vi "Open Form.vi"(8 "error in (no error)":errorcluster, 10 "Panel Form Controller":refnum<class "Panel Form Controller.lvclass">, 11 "Form Model in":refnum<class "Form Model.lvclass">) -> (0 "error out":errorcluster, 3 "Form Model out":refnum<class "Form Model.lvclass">)   [LabVIEW 2020, in "Form Model.lvlib" / "Form Model.lvclass"]
uses:
  Form Model.lvclass
  C:/Program Files (x86)/National Instruments/LabVIEW 2020/vi.lib/ActorFramework/Actor/Actor.lvclass
  Forms Controller/Form Controller/Panel Form Controller.lvclass
  <vilib>/ActorFramework/Actor/Actor.lvclass/Actor.ctl
  Form Model.lvclass/Form Model.ctl
  Forms Server/Form Server Messages Messages/Open Form Msg/Open Form Msg.lvclass/Open Form Msg.ctl
  <vilib>/ActorFramework/Message Enqueuer/Message Enqueuer.lvclass/Message Enqueuer.ctl
  <vilib>/ActorFramework/Message Enqueuer/Enqueue.vi
  Forms Server/Form Server Messages Messages/Open Form Msg/Open Form Msg.lvclass
  C:/Program Files (x86)/National Instruments/LabVIEW 2020/vi.lib/ActorFramework/Message/Message.lvclass
  <vilib>/ActorFramework/Message Priority Queue/Priority Enqueue.vi
  Form Model Configuration/Form Model Configuration Class/Form Model Configuration.lvclass
  Form Model Interfaces/Model Panel Logic Interface/Model Panel Logic.lvclass
  <vilib>/ActorFramework/Actor/Actor.lvclass
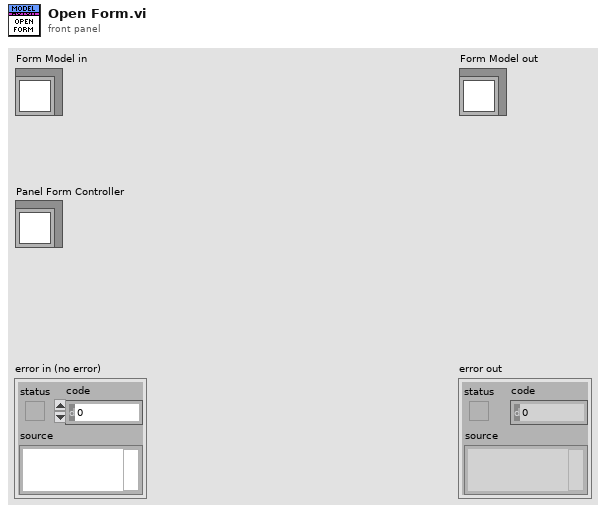
[diagram p1: front panel]
types:
  T1 = typedef "Form Server Interfaces.lvlib/Form ID.ctl" = cluster{"Name":string, "Panel type":string}
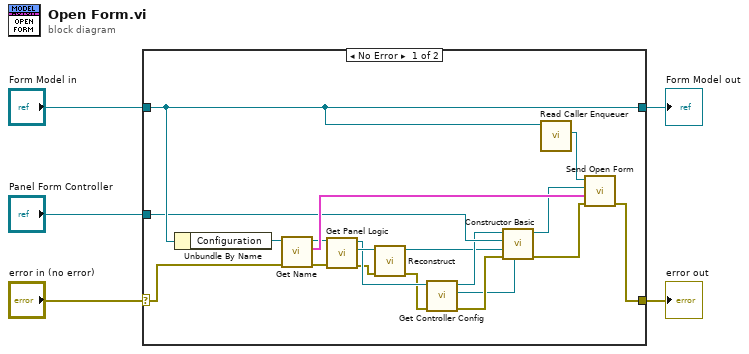
[diagram p0: block diagram]
diagram:
  n1 = case shown="No Error" "error in (no error)" {
    selector: "error in (no error)" -> [w15 w26]
    tunnel: "Form Model in" -> [w24 w25]
    tunnel: [w14 w26] -> w3
    tunnel: [w24 w25] -> w2
    tunnel: "Panel Form Controller" -> [w19 _]
    frame No Error {
      n2 = Unbundle By Name(w24) -> ("Configuration"=w22:refnum<class "Form Model Configuration.lvclass">)
      n3 = call-dynamic "Get Name.vi"("error in (no error)"=w15, "Form Configuration in"=w22) -> ("error out"=w11:errorcluster, "Form ID"=w21:T1, "Form Configuration out"=w12:refnum<class "Form Model Configuration.lvclass">)  [unwired: 7 in]
      n4 = call-dynamic "Get Panel Logic.vi"("error in (no error)"=w11, "Form Model Configuration in"=w12) -> ("error out"=w7:errorcluster, "Panel Logic"=w10:refnum<class "Model Panel Logic.lvclass">, "Form Model Configuration out"=w8:refnum<class "Form Model Configuration.lvclass">)  [unwired: 7 in]
      n5 = call-dynamic "Reconstruct.vi"("error in (no error)"=w7, "Model Panel Logic in"=w10) -> ("error out"=w6:errorcluster, "Model Panel Logic out"=w9:refnum<class "Model Panel Logic.lvclass">)  [unwired: 8 in]
      n6 = call-dynamic "Get Controller Config.vi"("error in (no error)"=w6, "Form Model Configuration in"=w8) -> ("error out"=w17:errorcluster, "Controller config"=w13:refnum<class "Panel Form Controller Configuration.lvclass">, "Form Model Configuration out"=w18:refnum<class "Form Model Configuration.lvclass">)  [unwired: 7 in]
      n7 = call "Constructor Basic.vi"("Controller Config"=w13, "error in (no error)"=w17, "Panel Logic"=w9, "Panel Form Controller"=w19, "Form Model Configuration in"=w18) -> ("error out"=w16:errorcluster, "Form Model Configuration out"=w20:refnum<class "Form Model Configuration.lvclass">)  [unwired: 5 in]
      n8 = call <vilib>:"Read Caller Enqueuer.vi"("Actor"=w24) -> ("Caller Enqueuer"=w23:refnum<class "Message Enqueuer.lvclass">)  [unwired: 10 in]
      n9 = call "Send Open Form.vi"("error in (no error)"=w16, "Caller Name"=w21, "Form Config"=w20, "Message Enqueuer"=w23) -> ("error out"=w14:errorcluster)  [unwired: 6 in, 1 out]
    }
    frame Error {
    }
  }
  "error out" <- w3
  "Form Model out" <- w2
